vi "createCommandList.vi"(8 "error in (no error)":errorcluster, 10 "Parameters":u32[](array[numeric]), 11 "Spannungseinbruch in":refnum<class "Spannungseinbruch.lvclass">) -> (0 "error out":errorcluster, 2 "Commandlist":string, 3 "Spannungseinbruch out":refnum<class "Spannungseinbruch.lvclass">)   [LabVIEW 2013, in "Spannungseinbruch.lvclass"]
uses:
  Spannungseinbruch.lvclass
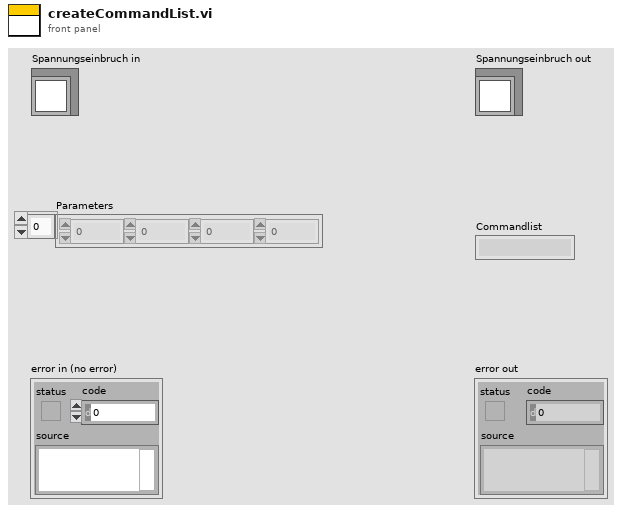
[diagram p1: front panel]
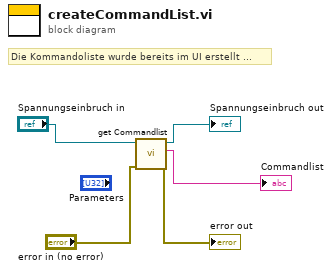
[diagram p0: block diagram]
diagram:
  # "Die Kommandoliste wurde bereits im UI erstellt ..."
  n1 = call-dynamic "get Commandlist.vi"("error in (no error)"="error in (no error)", "TestInterface (Eingang)"="Spannungseinbruch in") -> ("error out"=→"error out":errorcluster, "Commandlist"=→"Commandlist":string, "TestInterface (Ausgang)"=→"Spannungseinbruch out":refnum<class "Spannungseinbruch.lvclass">)  [unwired: 7 in]
